vi "incNoStepsAcq.vi"(2 "finPos":dbl, 3 "initPos":dbl, 4 "inp inc (mm)":dbl) -> (0 "no steps":i32, 1 "out inc (mm)":dbl=0.479232)   [LabVIEW 2015]
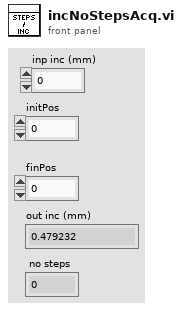
[diagram p1: front panel]
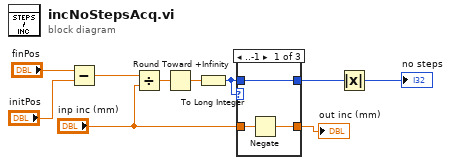
[diagram p0: block diagram]
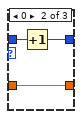
[diagram p2: hidden frame]
diagram:
  n1 = Subtract(x="finPos", y="initPos") -> (x-y=w8:dbl)
  n2 = Divide(x=w8, y="inp inc (mm)") -> (x/y=w9:dbl)
  n3 = Round Toward +Infinity(x=w9) -> (ceil(x): smallest int >= x=w2:dbl)
  n4 = To Long Integer(number=w2) -> (32bit integer=w1:i32)
  n5 = case shown="..-1" w1 {
    tunnel: w1 -> [w13 w16 w17]
    tunnel: [w13 w15 w17] -> w4
    tunnel: "inp inc (mm)" -> [w12 w14 w18]
    tunnel: [w11 w14 w18] -> w10
    frame ..-1 {
      n6 = Negate(x=w12) -> (-x=w11:dbl)
    }
    frame 0 {
      n7 = Increment(x=w16) -> (x+1=w15:i32)
    }
    frame 1.. {
    }
  }
  "out inc (mm)" <- w10
  n8 = Absolute Value(x=w4) -> (abs(x)=→"no steps":i32)
